vi "Get DAQ Settings.vi"(8 "error in (no error)":errorcluster, 11 "DAQ in":refnum<class "DAQ.lvclass">) -> (0 "error out":errorcluster, 2 "DAQ Settings":T1, 3 "DAQ out":refnum<class "DAQ.lvclass">)   [LabVIEW 2017, in "DAQ.lvclass"]
doc: "Developed by Kevin Thompson\nkevin@thompsonengineering.net\n\nCopyright 2018-2020\nThompson Engineering, LLC"
uses:
  DAQ.lvclass
  DataTypes/TD DAQ Settings--cluster.ctl
  DataTypes/TD DI Instrument Settings--cluster.ctl
  DataTypes/TD AI Instrument Settings--cluster.ctl
  DataTypes/TD AI InstSettings--cluster.ctl
  Process/ProcessSupport/TD SimAI Ranges--cluster.ctl
  DAQ.lvclass/DAQ.ctl
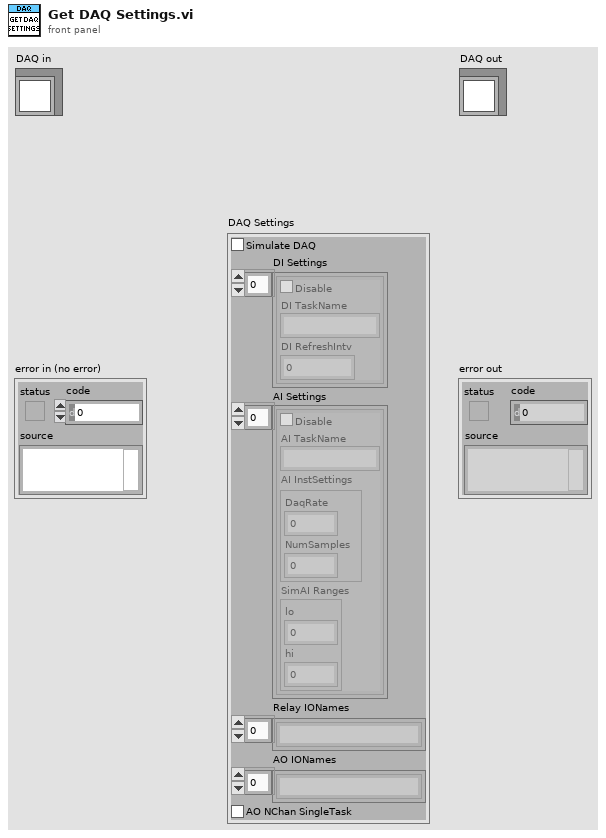
[diagram p1: front panel]
types:
  T1 = typedef "DAQ.lvclass/TD DAQ Settings--cluster.ctl" = cluster{"Simulate DAQ":bool, "DI Settings":T2[], "AI Settings":T3[], "Relay IONames":string[], "AO IONames":string[], "AO NChan SingleTask":bool}
  T2 = typedef "DAQ.lvclass/TD DI Instrument Settings--cluster.ctl" = cluster{"Disable":bool, "DI TaskName":string, "DI RefreshIntv":i32}
  T3 = typedef "DAQ.lvclass/TD AI Instrument Settings--cluster.ctl" = cluster{"Disable":bool, "AI TaskName":string, "AI InstSettings":T4, "SimAI Ranges":T5}
  T4 = typedef "DAQ.lvclass/TD AI InstSettings--cluster.ctl" = cluster{"DaqRate":dbl, "NumSamples":i32}
  T5 = typedef "DAQ.lvclass/TD SimAI Ranges--cluster.ctl" = cluster{"lo":dbl, "hi":dbl}
  T6 = typedef "DAQ.lvclass/TD Obj Data_DAQ--cluster.ctl" = cluster{"DAQ&TDMS State Data":T7, "DAQ Settings":T1, "DI TaskNames":string[], "AI TaskNames":string[], "DI IONames":string[], "DI SchemNames":string[], "DO IONames":string[], "DO SchemNames":string[], "AI IONames":string[], "AI SchemNames":string[], "AO IONames":string[], "AO SchemNames":string[]}
  T7 = typedef "DAQ.lvclass/TD DAQ&TDMS State Data--cluster.ctl" = cluster{"DAQState":T8, "vData":variant}
  T8 = typedef "DAQ.lvclass/TD DaqState--enum.ctl" = enum16{"Unknown", "Stopped", "Running", "Error"}
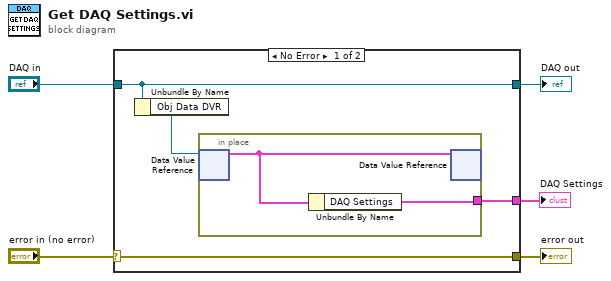
[diagram p0: block diagram]
diagram:
  n1 = case shown="No Error" "error in (no error)" {
    selector: "error in (no error)" -> [w9 w12]
    tunnel: [w9 w12] -> w4
    tunnel: [w8 w13] -> w2
    tunnel: "DAQ in" -> [w8 w13]
    tunnel: [w6 _] -> w1
    frame No Error {
      n2 = Unbundle By Name(w8) -> ("Obj Data DVR"=w7:refnum<data-value>)
      n3 = in-place {
        in-place-border: [w10] -> w6
        n4 = in-place-dvr #1(w7) -> (w11:T6)  [unwired: 1 out]
        n5 = Unbundle By Name(w11) -> ("DAQ Settings"=w10:T1)
        n6 = in-place-dvr #1(w11) -> ()  [unwired: 2 out]
      }
    }
    frame Error {
    }
  }
  "error out" <- w4
  "DAQ out" <- w2
  "DAQ Settings" <- w1
